vi "Read Configuration.vi"(8 "error in (no error)":errorcluster, 9 "Name (empty: type name)":string, 10 "Type":variant, 11 "ConfigurableActor in":refnum<class "ConfigurableActor.lvclass">) -> (0 "error out":errorcluster, 1 "any found?":bool, 2 "value":variant, 3 "ConfigurableActor out":refnum<class "ConfigurableActor.lvclass">, 4 "all found?":bool)   [LabVIEW 2014, in "ConfigurableActor.lvclass"]
uses:
  ConfigurableActor.lvclass
  ConfigurableActor.lvclass/ConfigurableActor.ctl
  <vilib>/LabVIEW Open Source/Configuration Manager/Manager/ConfigManager.lvclass/ConfigManager.ctl
  <vilib>/LabVIEW Open Source/Configuration Manager/Manager/Read.vi
  <vilib>/LabVIEW Open Source/Configuration Manager/Manager/Read Serializer.vi
  <vilib>/LabVIEW Open Source/Configuration Manager/Manager/Read Encoding.vi
  <vilib>/LabVIEW Open Source/Configuration Manager/Manager/Read Encryption.vi
  <vilib>/LabVIEW Open Source/Configuration Manager/Manager/Write.vi
  <vilib>/LabVIEW Open Source/Configuration Manager/Manager/Decompose KVPs.vi
  <vilib>/Utility/VariantDataType/GetTypeInfo.vi
  <vilib>/LabVIEW Open Source/Data Manipulation/KVP Parser.vi
  <vilib>/LabVIEW Open Source/Configuration Manager/Cache/ConfigManager.Cache.lvclass
  <vilib>/LabVIEW Open Source/Configuration Manager/Manager/ConfigManager.lvclass
  <vilib>/LabVIEW Open Source/Configuration Manager/Encoding/Encoding.lvclass
  <vilib>/LabVIEW Open Source/Configuration Manager/Encryption/Encryption.lvclass
  <vilib>/LabVIEW Open Source/Configuration Manager/Serializer/Serializer.lvclass
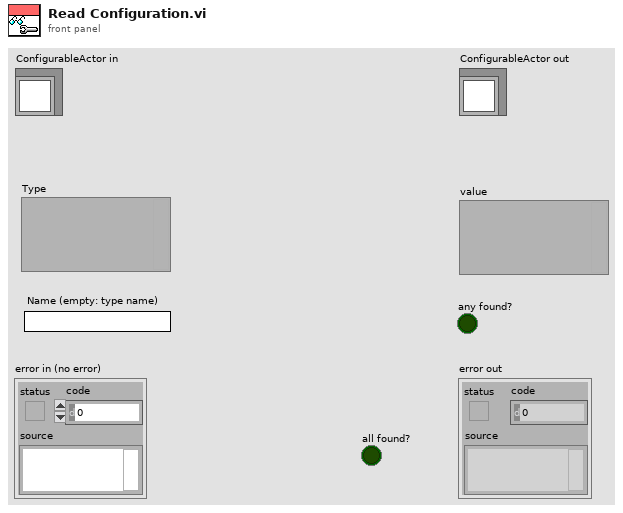
[diagram p1: front panel]
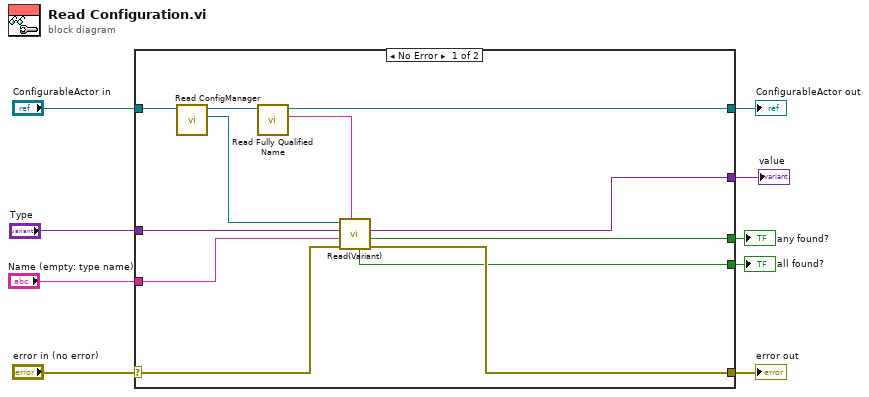
[diagram p0: block diagram]
diagram:
  n1 = case shown="No Error" "error in (no error)" {
    selector: "error in (no error)" -> [w16 w23]
    tunnel: [w15 w23] -> w8
    tunnel: [w19 w22] -> w6
    tunnel: "ConfigurableActor in" -> [w21 w22]
    tunnel: [w14 _] -> w5
    tunnel: [w13 _] -> w4
    tunnel: [w12 _] -> w1
    tunnel: "Type" -> [w11 _]
    tunnel: "Name (empty: type name)" -> [w10 _]
    frame No Error {
      n2 = call "Read ConfigManager.vi"("ConfigurableActor in"=w21) -> ("ConfigManager"=w18:refnum<class "ConfigManager.lvclass">, "ConfigurableActor out"=w20:refnum<class "ConfigurableActor.lvclass">)  [unwired: 8 in, 1 out]
      n3 = call "Read Fully Qualified Name.vi"("ConfigurableActor in"=w20) -> ("Fully Qualified Name"=w17:string, "ConfigurableActor out"=w19:refnum<class "ConfigurableActor.lvclass">)  [unwired: 8 in, 1 out]
      n4 = call <vilib>:"Read(Variant).vi"("Qualified Name"=w17, "error in (no error)"=w16, "Name (empty: type name)"=w10, "Type"=w11, "ConfigManager in"=w18) -> ("error out"=w15:errorcluster, "any found?"=w14:bool, "value"=w12:variant, "all found?"=w13:bool)  [unwired: 2 in, 1 out]
    }
    frame Error {
    }
  }
  "error out" <- w8
  "ConfigurableActor out" <- w6
  "any found?" <- w5
  "all found?" <- w4
  "value" <- w1
